vi "FGV SAE J-1939 Test Data Environment.vi"(6 "Aktion":T2(ring), 8 "Test Modus":bool, 9 "LogFileParameter":T1={"Group Name"="DAF", "Channel Name"="My Channel", "Anzahl Testdaten"=-1}, 10 "SAE J-1939 Log Datei":path=path "E:/LabVIEW/2020/CanBus_OFS/OBD/TU Graz DAF SAEJ1939/Test TU Graz DAF/DAF3.tdms", 11 "Offset Frame ID":i32=-2) -> (0 "Test Modus":bool, 1 "LogFileParameter":T1, 2 "SAE J-1939 Log Datei":path, 3 "Offset Frame ID":i32)   [LabVIEW 2020, in "CAN Konfig.lvlib"]
uses:
  CAN Konfig.lvlib
  Allgemein/allgemeine Sub-VIs.lvlib
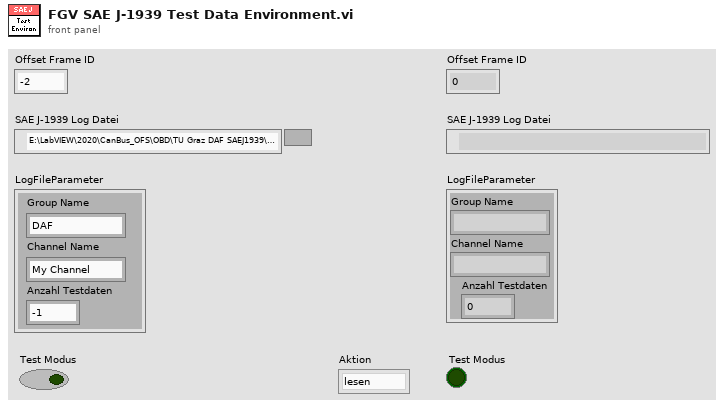
[diagram p1: front panel]
types:
  T1 = cluster{"Group Name":string, "Channel Name":string, "Anzahl Testdaten":i32}
  T2 = enum16{"lesen", "schreiben", "laden", "speichern"}
  T3 = enum16{"open", "replace", "create", "open or create", "replace or create", "replace or create with confirmation"}
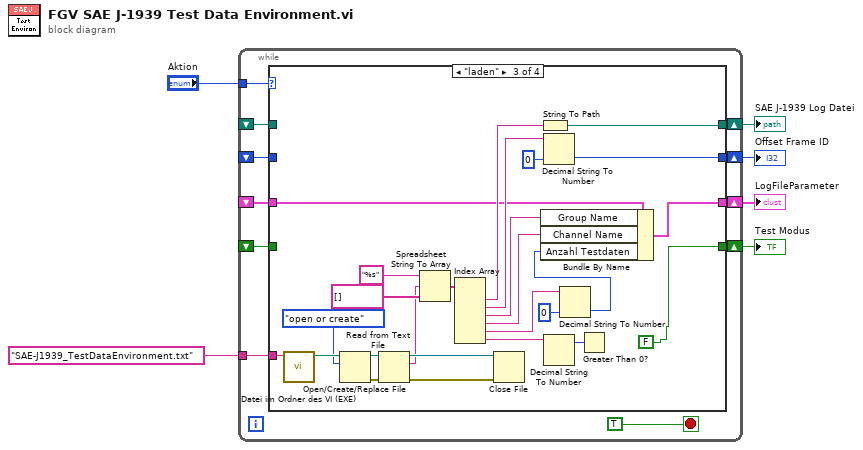
[diagram p0: block diagram]
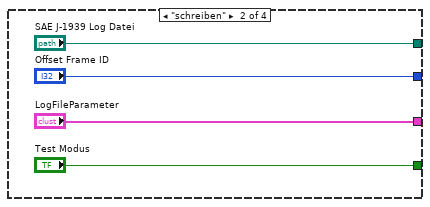
[diagram p3: hidden frame]
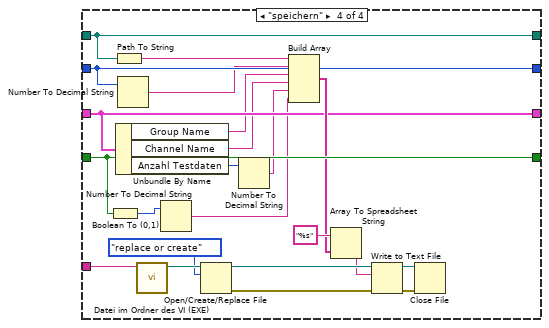
[diagram p4: hidden frame]
diagram:
  n1 = while {
    tunnel: "Aktion" -> [w16]
    shift-right: [w15] -> w5
    shift-left: _ -> [w12]
    shift-right: [w14] -> w4
    shift-left: _ -> [w11]
    shift-right: [w13] -> w3
    shift-left: _ -> [w10]
    tunnel: "SAE-J1939_TestDataEnvironment.txt" ("Dateiname") -> [w9]
    shift-right: [w8] -> w1
    shift-left: _ -> [w7]
    stop <- TRUE stop-if-true
    n2 = case shown="\"laden\"" w16 {
      tunnel: [w21 "SAE J-1939 Log Datei" w40 w67] -> w15
      tunnel: [w20 "Offset Frame ID" w36 w65] -> w14
      tunnel: [w19 "Test Modus" FALSE ("Test Modus") w64] -> w13
      tunnel: w12 -> [w21 _ _ w67]
      tunnel: w11 -> [w20 _ _ w65]
      tunnel: w10 -> [w19 _ _ w64]
      tunnel: w9 -> [_ _ w51 w73]
      tunnel: [w18 "LogFileParameter" w30 w57] -> w8
      tunnel: w7 -> [w18 _ w33 w57]
      frame "lesen", Default {
      }
      frame "schreiben" {
      }
      frame "laden" {
        n3 = call "Datei im Ordner des VI (EXE).vi"("Dateiname"=w51) -> ("Dateipfad im Ordner des Haupt-VIs"=w46:path)  [unwired: 8 in, 2 out]
        n4 = Open/Create/Replace File(file path (use dialog)=w46, operation (0:open)=T3."open or create" ("Operation (0:open)")) -> (refnum out=w48:refnum<file>, error out=w47:errorcluster)  [unwired: 4 in, 1 out]
        n5 = Read from Text File(file (use dialog)=w48, error in=w47) -> (refnum out=w50:refnum<file>, text=w42:string, error out=w49:errorcluster)  [unwired: 3 out]
        n6 = Spreadsheet String To Array(format string="%s" ("Format-String"), spreadsheet string=w42, array type (2D Dbl)=string[] []) -> (array=w41:string[])  [unwired: 1 out]
        n7 = Index Array(array=w41) -> (element #1=w39:string, element #2=w38:string, element #3=w29:string, element #4=w28:string, element #5=w31:string, element #6=w32:string)  [unwired: 6 in]
        n8 = Close File(refnum=w50, error in=w49) -> ()  [unwired: 2 out]
        n9 = String To Path(string=w39) -> (path=w40:path)
        n10 = Decimal String To Number(string=w38, default (0L)=0 ("Standard (0 I32)")) -> (number=w36:i32)  [unwired: 1 in, 1 out]
        n11 = Decimal String To Number(string=w32) -> (offset past number=w37:i32)  [unwired: 2 in, 1 out]
        n12 = Decimal String To Number(string=w31, default (0L)=0 ("Standard (0 I32)")) -> (number=w27:i32)  [unwired: 1 in, 1 out]
        n13 = Bundle By Name(cluster=w33, "Group Name"=w29, "Channel Name"=w28, "Anzahl Testdaten"=w27) -> (w30:T1)
        n14 = Greater Than 0?(x=w37) -> ()  [unwired: 1 out]
      }
      frame "speichern" {
        n15 = Boolean To (0,1)(Boolean=w64) -> (0, 1=w63:i16)
        n16 = Path To String(path=w67) -> (string=w62:string)
        n17 = Unbundle By Name(w57) -> ("Group Name"=w55:string, "Channel Name"=w54:string, "Anzahl Testdaten"=w56:i32)
        n18 = Number To Decimal String(number=w65) -> (decimal integer string=w58:string)  [unwired: 1 in]
        n19 = call "Datei im Ordner des VI (EXE).vi"("Dateiname"=w73) -> ("Dateipfad im Ordner des Haupt-VIs"=w68:path)  [unwired: 8 in, 2 out]
        n20 = Number To Decimal String(number=w63) -> (decimal integer string=w52:string)  [unwired: 1 in]
        n21 = Open/Create/Replace File(file path (use dialog)=w68, operation (0:open)=T3."replace or create" ("Operation (0:open)")) -> (refnum out=w69:refnum<file>, error out=w70:errorcluster)  [unwired: 4 in, 1 out]
        n22 = Number To Decimal String(number=w56) -> (decimal integer string=w53:string)  [unwired: 1 in]
        n23 = Build Array(w62, w58, w55, w54, w53, w52) -> (w60:string[])
        n24 = Array To Spreadsheet String(array=w60, 3:"%s" ("Format-String")) -> (spreadsheet string=w59:string)  [unwired: 1 in]
        n25 = Write to Text File(file (use dialog)=w69, text=w59, error in=w70) -> (refnum out=w72:refnum<file>, error out=w71:errorcluster)  [unwired: 1 in, 1 out]
        n26 = Close File(refnum=w72, error in=w71) -> ()  [unwired: 2 out]
      }
    }
  }
  "SAE J-1939 Log Datei" <- w5
  "Offset Frame ID" <- w4
  "Test Modus" <- w3
  "LogFileParameter" <- w1
